vi "SHOWCASEVERSION.vi"() -> ()   [LabVIEW 2024]
uses:
  <vilib>/Utility/file.llb/Read Delimited Spreadsheet (DBL).vi
panel:
  in  "Flow Rate Lower Limit 2":dbl
  in  "Flow Rate Upper Limit 2":dbl
  in  "Desired Flow Rate 3":dbl format="%_2f"
  in  "Initial RPM  3":dbl format="%_4f"
  in  "stop 2":bool
  out "Boolean":bool
  out "Waveform Chart 3":dbl[](graph)
  out "Waveform Chart 2":dbl(graph)
  out "Flow Rate":dbl(graph)
  in  "Color Box":u32(colorbox)
  # "Blood Flow Rate"
  # "Flow Rate (mL/min)"
  # "Initial LVAD Speed (RPM)"
  # "Desired Flow Rate (mL/min)"
  # "LVAD Speed"
  # "Upper Flow Rate Limit (mL/min)"
  # "Speed (RPM)"
  # "Lower Flow Rate Limit (mL/min)"
  # "Optimal Flow State"
  # "Right Heart Waveform"
  # "Amplitude"
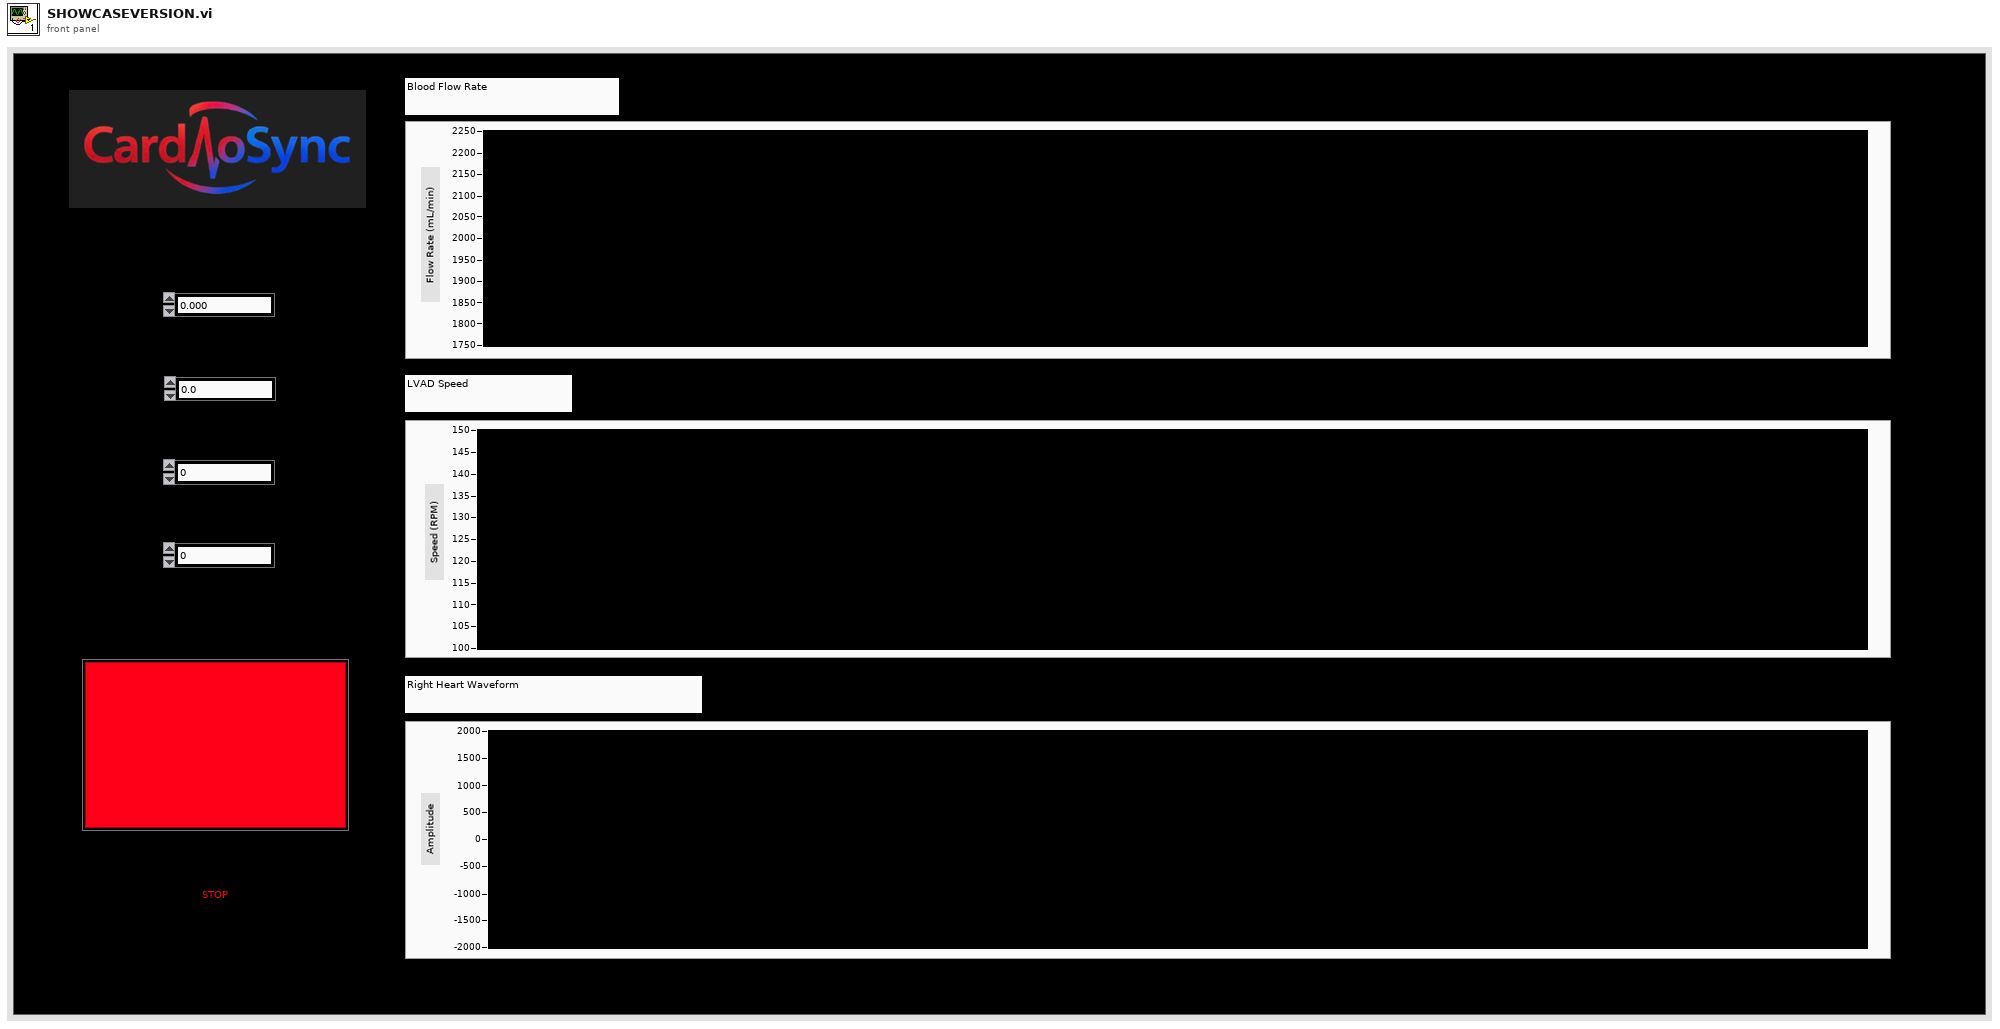
[diagram p1: front panel]
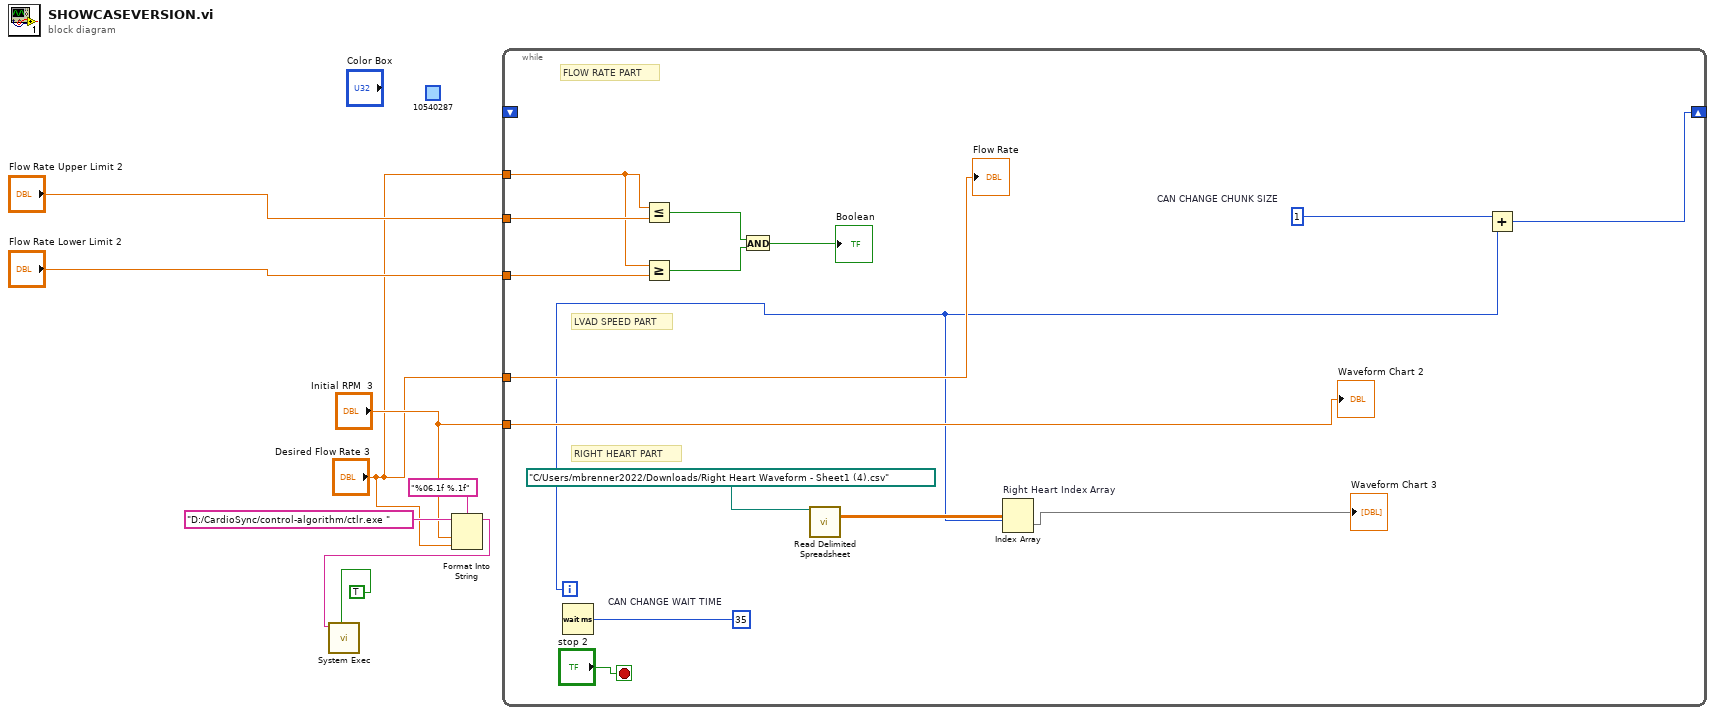
[diagram p0: block diagram]
diagram:
  (unwired) u32 10540287 ("Color Box 2")
  n1 = Format Into String(format string="%06.1f %.1f", initial string="D:/CardioSync/control-algorithm/ctlr.exe ", "Initial RPM  3", "Desired Flow Rate 3") -> (resulting string=w4:string)  [unwired: 1 in, 1 out]
  n2 = call <vilib>:"System Exec.vi"("wait until completion? (T)"=TRUE, "command line"=w4) -> ()  [unwired: 6 in, 4 out]
  n3 = while {
    shift-right: [w23] -> _
    shift-left: _ -> [_]
    tunnel: "Flow Rate Upper Limit 2" -> [w15]
    tunnel: "Flow Rate Lower Limit 2" -> [w14]
    tunnel: "Desired Flow Rate 3" -> [w12]
    tunnel: "Initial RPM  3" -> [w13]
    tunnel: "Desired Flow Rate 3" -> [w11]
    i -> [w9]
    stop <- "stop 2" stop-if-true
    w24 = u32 35  # CAN CHANGE WAIT TIME
    w21 = 1  # CAN CHANGE CHUNK SIZE
    # "RIGHT HEART PART"
    # "LVAD SPEED PART"
    # "FLOW RATE PART"
    n4 = Wait (ms)(milliseconds to wait=w24) -> ()  [unwired: 1 out]
    n5 = Less Or Equal?(x=w12, y=w15) -> (x <= y?=w19:bool)
    n6 = Greater Or Equal?(x=w12, y=w14) -> (x >= y?=w18:bool)
    n7 = And(x=w19, y=w18) -> (x .and. y?=→"Boolean":bool)
    n8 = call-poly <vilib>:"Read Delimited Spreadsheet.vi"("file path (dialog if empty)"=path "C:/Users/mbrenner2022/Downloads/Right Heart Waveform - Sheet1 (4).csv") -> ("all rows"=w22:dbl[][])  [unwired: 9 in, 5 out]
    n9 = Index Array "Right Heart Index Array"(array=w22, index (row)=w9) -> (element=→"Waveform Chart 3":dbl[])  [unwired: 1 in]
    n10 = Add(x=w21, y=w9) -> (x+y=w23:i32)
    "Waveform Chart 2" <- w13
    "Flow Rate" <- w11
  }
